vi "set_frequencies.vi"(8 "error in (no error)":errorcluster, 9 "AOD bandwidth freq. (Hz)":dbl[unit], 10 "AOD center freq. (Hz)":dbl[unit], 11 "FPGAWrapperMH120124RAPS_PXI7813R in":refnum<class "FPGAWrapperMH120124RAPS_PXI7813R.lvclass">) -> (0 "error out":errorcluster, 3 "FPGAWrapperMH120124RAPS_PXI7813R out":refnum<class "FPGAWrapperMH120124RAPS_PXI7813R.lvclass">)   [LabVIEW 2010, in "FPGAWrapperMH120124RAPS_PXI7813R.lvclass"]
uses:
  FPGAWrapperMH120124RAPS_PXI7813R.lvclass
  FPGAWrapperMH120124RAPS_PXI7813R.lvclass/FPGAWrapperMH120124RAPS_PXI7813R.ctl
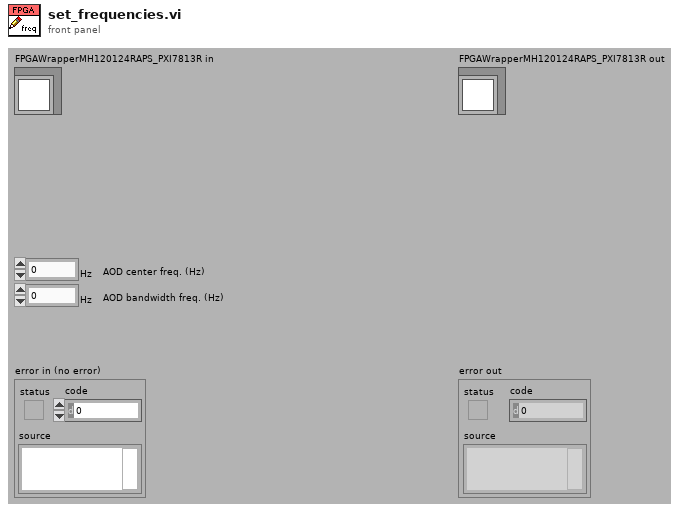
[diagram p1: front panel]
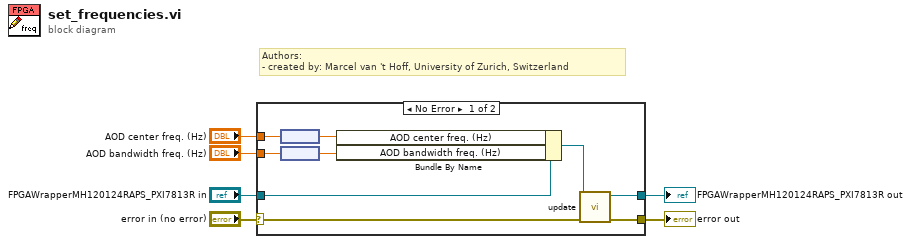
[diagram p0: block diagram]
diagram:
  # "Authors: \n- created by: Marcel van 't Hoff, University of Zurich, Switzerland"
  n1 = case shown="No Error" "error in (no error)" {
    selector: "error in (no error)" -> [w10 w16]
    tunnel: [w9 w16] -> w3
    tunnel: [w8 w17] -> w5
    tunnel: "FPGAWrapperMH120124RAPS_PXI7813R in" -> [w15 w17]
    tunnel: "AOD center freq. (Hz)" -> [w14 _]
    tunnel: "AOD bandwidth freq. (Hz)" -> [w12 _]
    frame No Error {
      n2 = node(w14) -> (w13:dbl)
      n3 = node(w12) -> (w11:dbl)
      n4 = Bundle By Name(cluster=w15, "AOD center freq. (Hz)"=w13, "AOD bandwidth freq. (Hz)"=w11) -> (w7:refnum<class "FPGAWrapperMH120124RAPS_PXI7813R.lvclass">)
      n5 = call-dynamic "update.vi"("error in (no error)"=w10, "FPGAWrapperMH120124RAPS_PXI7813R in"=w7) -> ("error out"=w9:errorcluster, "FPGAWrapperMH120124RAPS_PXI7813R out"=w8:refnum<class "FPGAWrapperMH120124RAPS_PXI7813R.lvclass">)  [unwired: 8 in]
    }
    frame Error {
    }
  }
  "error out" <- w3
  "FPGAWrapperMH120124RAPS_PXI7813R out" <- w5
